vi "hasStopped.vi"(8 "error in (no error)":errorcluster, 10 "stoppedByUser":bool, 11 "ExperimentControlEvents in":refnum<class "ExperimentControlEvents.lvclass">) -> (0 "error out":errorcluster, 3 "ExperimentControlEvents out":refnum<class "ExperimentControlEvents.lvclass">)   [LabVIEW 2011, in "Views.lvlib" / "ExperimentControl.lvlib" / "ExperimentControlEvents.lvclass"]
uses:
  ExperimentControlEvents.lvclass
  ExperimentControlEvents.lvclass/ExperimentControlEvents.ctl
  Events/Event.lvclass
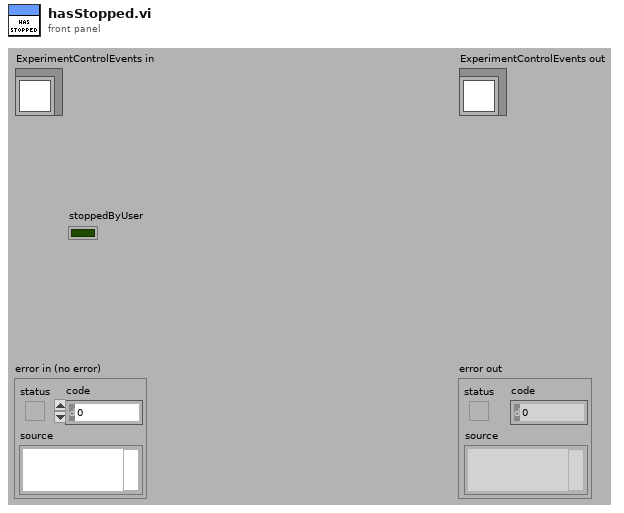
[diagram p1: front panel]
types:
  T1 = enum16{"close", "stopRunning", "runSingleScript", "runExperiment", "runExperimentScript", "Unregistered", "hasStopped"}
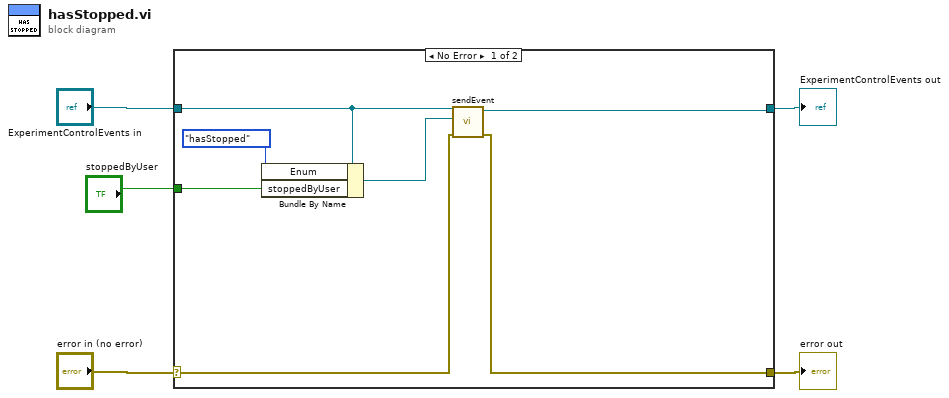
[diagram p0: block diagram]
diagram:
  n1 = case shown="No Error" "error in (no error)" {
    selector: "error in (no error)" -> [w9 w14]
    tunnel: [w8 w14] -> w2
    tunnel: [w12 w13] -> w5
    tunnel: "ExperimentControlEvents in" -> [w11 w13]
    tunnel: "stoppedByUser" -> [w6 _]
    frame No Error {
      n2 = Bundle By Name(cluster=w11, "Enum"=T1."hasStopped", "stoppedByUser"=w6) -> (w10:refnum<class "ExperimentControlEvents.lvclass">)
      n3 = call "sendEvent.vi"("error in (no error)"=w9, "data"=w10, "Event in"=w11) -> ("error out"=w8:errorcluster, "Event out"=w12:refnum<class "ExperimentControlEvents.lvclass">)  [unwired: 7 in]
    }
    frame Error {
    }
  }
  "error out" <- w2
  "ExperimentControlEvents out" <- w5
